vi "WCA_GET_YTO_COARSE_TUNE.vi"(0 "Cartridge Band":u32=10, 1 "Slave Node in":cluster{"Address":i16, "Serial Number":i8[]}={"Address"=19, "Serial Number"=[16, 71, 55, 76, 1, 8, 0, -15]} {"Serial Number" format="%.0x"; "Address" format="%.0x"}, 2 "ObjHandle in":u32, 11 "error in (no error)":errorcluster) -> (4 "ObjHandle out":u32=92930112, 8 "GET_YTO_COARSE_TUNE":u16, 15 "error out":errorcluster)   [LabVIEW 2017]
uses:
  WCA_Global.vi
panel:
  # "Node Address"
  # "Serial Number"
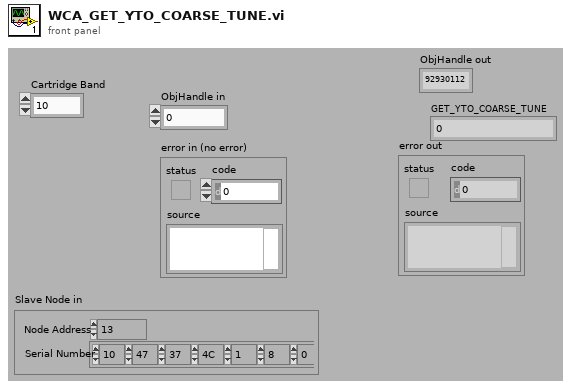
[diagram p1: front panel]
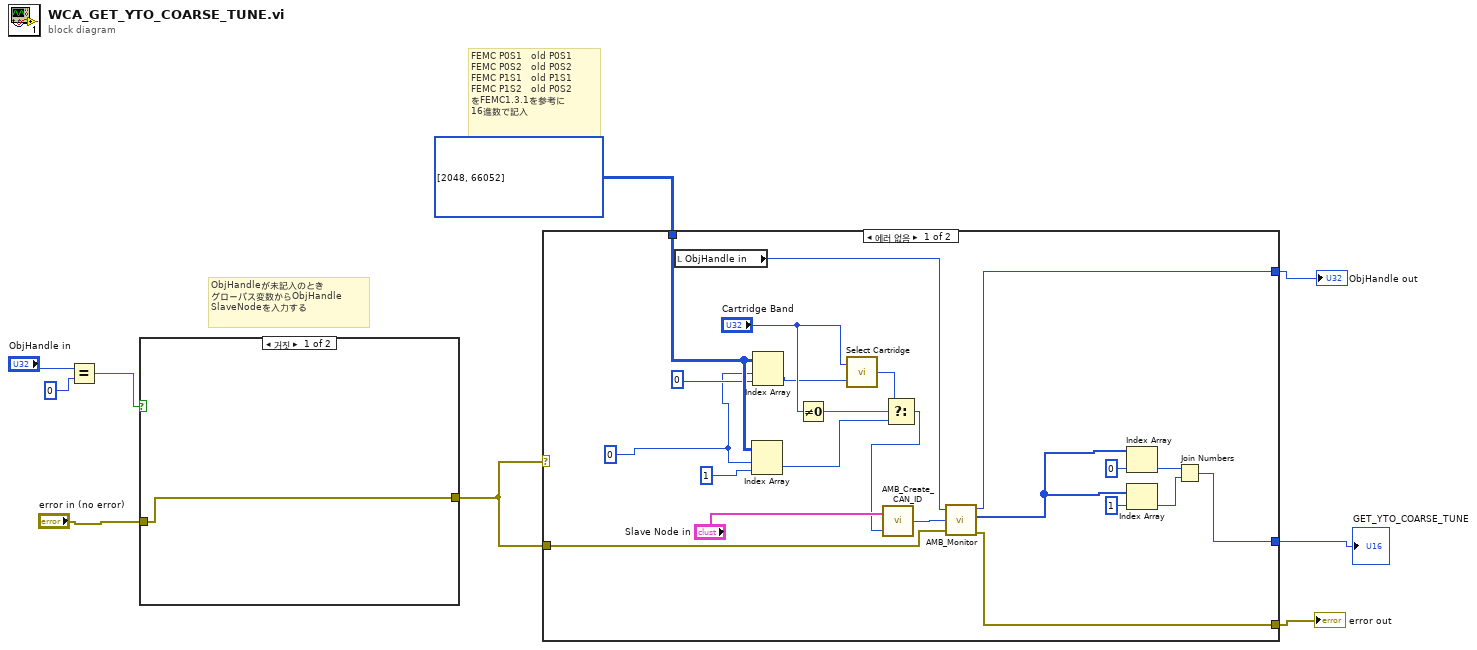
[diagram p0: block diagram]
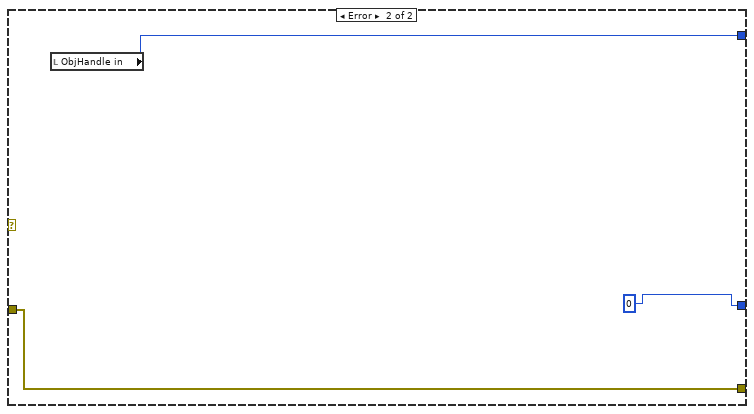
[diagram p2: hidden frame]
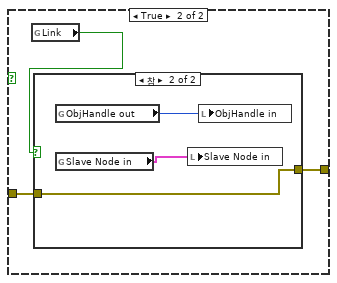
[diagram p3: hidden frame]
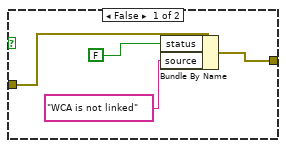
[diagram p4: hidden frame]
diagram:
  # "ObjHandleが未記入のとき\nグローバス変数からObjHandle\nSlaveNodeを入力する"
  # "FEMC P0S1   old P0S1\nFEMC P0S2   old P0S2\nFEMC P1S1   old P1S1\nFEMC P1S2   old P0S2\nをFEMC1.3.1を参考に\n16進数で記入"
  n1 = Equal?(x="ObjHandle in", y=0) -> (x = y?=w7:bool)
  n2 = case shown="거짓" w7 {
    tunnel: "error in (no error)" -> [w10 w13]
    tunnel: [w10 w12] -> w5
    frame False {
    }
    frame True {
      n3 = global read "WCA_Global.vi" "Link"() -> (w11:bool)
      n4 = case shown="참" w11 {
        tunnel: w13 -> [w17 w18]
        tunnel: [w14 w18] -> w12
        frame False {
          n5 = Bundle By Name(cluster=w17, "status"=FALSE, "source"="WCA is not linked") -> (w14:errorcluster)
        }
        frame True {
          n6 = global read "WCA_Global.vi" "ObjHandle out"() -> (w20:u32)
          n7 = global read "WCA_Global.vi" "Slave Node in"() -> (w19:cluster{"Address":i16, "Serial Number":i8[]})
          n8 = local write "Slave Node in"(w19) -> ()
          n9 = local write "ObjHandle in"(w20) -> ()
        }
      }
    }
  }
  n10 = case shown="에러 없음" w5 {
    tunnel: w5 -> [w29 w45]
    tunnel: [w30 w44] -> w4
    tunnel: [w28 w45] -> w3
    tunnel: i32[][] [[2048, 66052]] -> [w42 _]
    tunnel: [w23 0] -> w1
    frame No Error {
      w27 = 0
      n11 = local read "ObjHandle in"() -> (w31:u32)
      n12 = Index Array(array=w42, index (row)=w27, index (col)=1) -> (element=w38:i32)
      n13 = Index Array(array=w42, index (row)=w27, index (col)=0) -> (element=w37:i32)
      n14 = Not Equal To 0?(x="Cartridge Band") -> (x != 0?=w40:bool)
      n15 = call "Select Cartridge.vi"("Relative Address in"=w37, "Cartridge band"="Cartridge Band") -> ("Relative Address out"=w41:u32)
      n16 = Select(t=w41, s=w40, f=w38) -> (s? t:f=w32:u32)
      n17 = call "AMB_Create_CAN_ID.vi"("Relative Address in"=w32, "Slave Node in"="Slave Node in") -> ("CAN ID out"=w34:u32)
      n18 = call "AMB_Monitor.vi"("ObjHandle in"=w31, "CAN ID in"=w34, "error in"=w29) -> ("ObjHandle out"=w30:u32, "Data Array out"=w24:u8[], "error out"=w28:errorcluster)  [unwired: 1 out]
      n19 = Index Array(array=w24, index=0) -> (element=w22:u8)
      n20 = Index Array(array=w24, index=1) -> (element=w21:u8)
      n21 = Join Numbers(hi=w22, lo=w21) -> ((hi.lo)=w23:u16)
    }
    frame Error {
      n22 = local read "ObjHandle in"() -> (w44:u32)
    }
  }
  "ObjHandle out" <- w4
  "error out" <- w3
  "GET_YTO_COARSE_TUNE" <- w1
